vi "Calculate Axis Cluster.vi"(6 "Justify":enum16{"Start", "Center", "End"}(ring), 10 "Step Size":dbl, 11 "X Axis in":T1) -> (3 "X Axis out":T1)   [LabVIEW 2017]
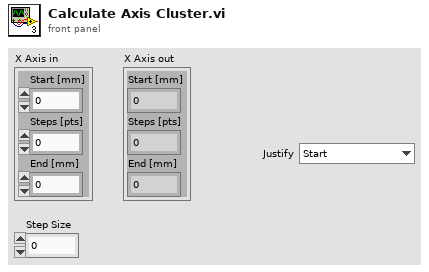
[diagram p1: front panel]
types:
  T1 = cluster{"Start [mm]":dbl, "Steps [pts]":u16, "End [mm]":dbl}
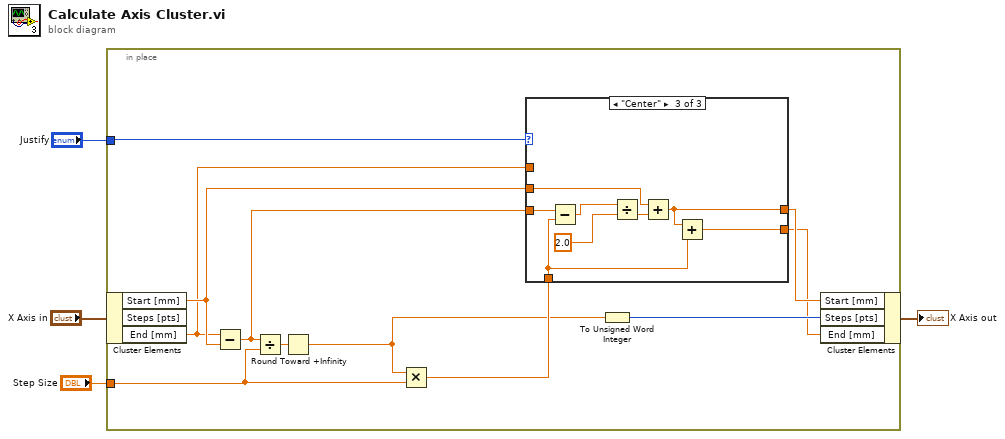
[diagram p0: block diagram]
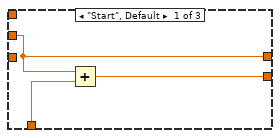
[diagram p2: hidden frame]
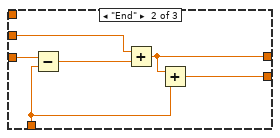
[diagram p3: hidden frame]
diagram:
  n1 = in-place {
    in-place-border: "Step Size" -> [w13]
    in-place-border: "Justify" -> [w12]
    n2 = in-place-cluster #1("X Axis in") -> ("Start [mm]"=w11:dbl, "End [mm]"=w10:dbl)  [unwired: 1 out]
    n3 = Subtract(x=w10, y=w11) -> (x-y=w8:dbl)
    n4 = Divide(x=w8, y=w13) -> (x/y=w15:dbl)
    n5 = Round Toward +Infinity(x=w15) -> (ceil(x): smallest int >= x=w5:dbl)
    n6 = Multiply(x=w5, y=w13) -> (x*y=w9:dbl)
    n7 = case shown="\"Center\"" w12 {
      tunnel: w11 -> [w17 w22 w30]
      tunnel: w10 -> [_ _ _]
      tunnel: [w16 w20 w25] -> w6
      tunnel: [w17 w19 w26] -> w7
      tunnel: w9 -> [w18 w21 w29]
      tunnel: w8 -> [_ w24 w32]
      frame "Start", Default {
        n8 = Add(x=w17, y=w18) -> (x+y=w16:dbl)
      }
      frame "End" {
        n9 = Subtract(x=w24, y=w21) -> (x-y=w23:dbl)
        n10 = Add(x=w22, y=w23) -> (x+y=w19:dbl)
        n11 = Add(x=w19, y=w21) -> (x+y=w20:dbl)
      }
      frame "Center" {
        n12 = Subtract(x=w32, y=w29) -> (x-y=w31:dbl)
        n13 = Divide(x=w31, y=2.0 ("x")) -> (x/y=w28:dbl)
        n14 = Add(x=w30, y=w28) -> (x+y=w26:dbl)
        n15 = Add(x=w26, y=w29) -> (x+y=w25:dbl)
      }
    }
    n16 = To Unsigned Word Integer(number=w5) -> (unsigned 16bit integer=w14:u16)
    n17 = in-place-cluster #1("Start [mm]"=w7, "Steps [pts]"=w14, "End [mm]"=w6) -> (→"X Axis out":T1)
  }
